vi "create_gcs.vi"(10 "Path":string) -> (3 "source":refnum<class "gcs.lvclass">)   [LabVIEW 2020, in "datasources.lvlib" / "source.lvclass"]
uses:
  source.lvclass/source.ctl
  path.set.vi
  source.lvclass
  gcs/gcs.lvclass
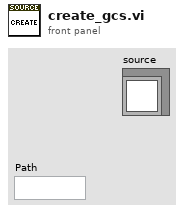
[diagram p1: front panel]
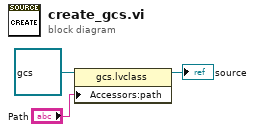
[diagram p0: block diagram]
diagram:
  n1 = property class="gcs.lvclass"(reference=refnum<class "gcs.lvclass"> refnum ("datasources.lvlib:gcs.lvclass"), "Accessors:path"="Path") -> (reference out=→"source":refnum<class "gcs.lvclass">)  [unwired: 1 in, 1 out]
